vi "Next Bind.vi"(8 "error in (no error)":errorcluster, 10 "Next Bind":i32, 11 "SQL Statement in":refnum<class "SQL Statement.lvclass">) -> (0 "error out":errorcluster, 3 "SQL Statement out":refnum<class "SQL Statement.lvclass">)   [LabVIEW 2013, in "SQLiteSupport.lvlib" / "SQL Statement.lvclass"]
doc: "Sets the index of the next parameter to be bound. Note that this index self-increments with each Bind, so it is optional to actually explicitly set the next bind."
uses:
  SQL Statement.lvclass
  SQL Statement.lvclass/SQL Statement.ctl
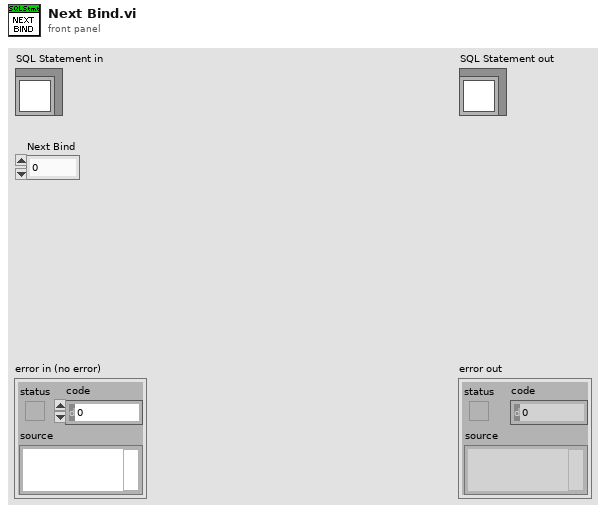
[diagram p1: front panel]
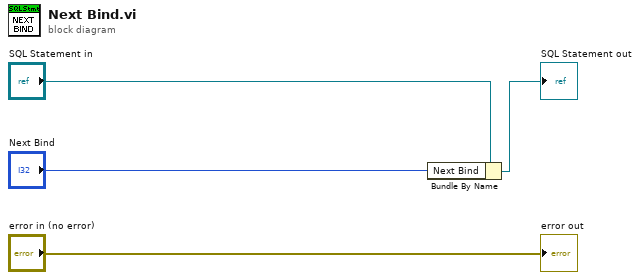
[diagram p0: block diagram]
diagram:
  n1 = Bundle By Name(cluster="SQL Statement in", "Next Bind"="Next Bind") -> (→"SQL Statement out":refnum<class "SQL Statement.lvclass">)
  "error out" <- "error in (no error)"
